vi "PID Setpoint Profile.vi"(4 "reinitialize? (F)":bool, 6 "dt (s)":dbl=-1.0 format="%.3f", 9 "setpoint profile":cluster{"time (s)":dbl, "setpoint":dbl}[](array[cluster]) {"setpoint" format="%.2f"; "time (s)" format="%.3f"}) -> (0 "dt out (s)":dbl format="%.3f", 1 "elapsed time (s)":dbl format="%.3f", 2 "profile complete?":bool, 3 "setpoint":dbl format="%.2f")   [LabVIEW 2017, in "NI_PID_pid.lvlib"]
doc: "Generates setpoint values over time in a control loop for ramp and soak types of control applications."
uses:
  <vilib>/addons/control/pid/NI_PID_pid.lvlib
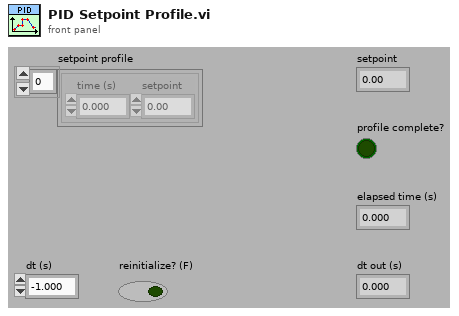
[diagram p1: front panel]
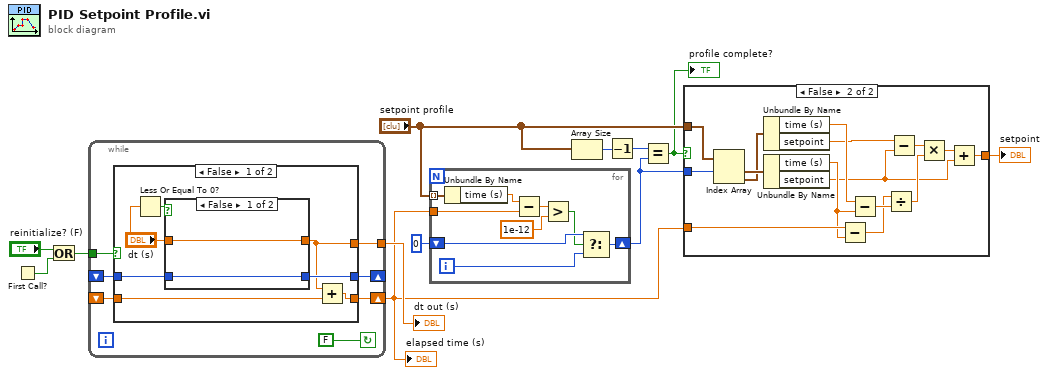
[diagram p0: block diagram]
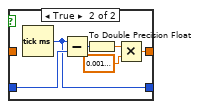
[diagram p2: hidden frame]
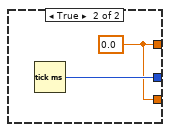
[diagram p3: hidden frame]
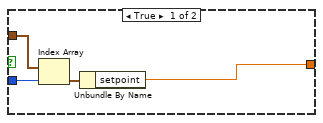
[diagram p4: hidden frame]
diagram:
  n1 = First Call?() -> (First Call?: T/F=w12:bool)
  n2 = Or(x="reinitialize? (F)", y=w12) -> (x .or. y?=w11:bool)
  n3 = while {
    tunnel: [w13] -> w2
    shift-left: _ -> [w16]
    shift-right: [w17] -> w1
    tunnel: w11 -> [w19]
    shift-left: _ -> [w14]
    shift-right: [w18] -> _
    stop <- FALSE continue-if-true
    n4 = case shown="False" w19 {
      tunnel: [w21 w36] -> w18
      tunnel: [w26 w35] -> w17
      tunnel: w16 -> [w25 _]
      tunnel: w14 -> [w22 _]
      tunnel: [w20 w35] -> w13
      frame False {
        n5 = Less Or Equal To 0?(x="dt (s)") -> (x <= 0?=w24:bool)
        n6 = case shown="False" w24 {
          tunnel: [w28 w31] -> w20
          tunnel: w22 -> [w27 w30]
          tunnel: [w27 w29] -> w21
          tunnel: "dt (s)" -> [w28 _]
          frame False {
          }
          frame True {
            n7 = Tick Count (ms)() -> (millisecond timer value=w29:u32)
            n8 = Subtract(x=w29, y=w30) -> (x-y=w33:u32)
            n9 = To Double Precision Float(number=w33) -> (double precision float=w32:dbl)
            n10 = Multiply(x=w32, y=0.0010000000474974513) -> (x*y=w31:dbl)
          }
        }
        n11 = Add(x=w20, y=w25) -> (x+y=w26:dbl)
      }
      frame True {
        w35 = 0.0
        n12 = Tick Count (ms)() -> (millisecond timer value=w36:u32)
      }
    }
  }
  "dt out (s)" <- w2
  "elapsed time (s)" <- w1
  n13 = for {
    tunnel: "setpoint profile" -> [w45] mode=indexing
    tunnel: w1 -> [w42]
    shift-right: [w44] -> w7
    shift-left: 0 -> [w41]
    i -> [w40]
    n14 = Unbundle By Name(w45) -> ("time (s)"=w43:dbl)
    n15 = Subtract(x=w43, y=w42) -> (x-y=w38:dbl)
    n16 = Greater?(x=w38, y=1e-12) -> (0:w39:bool)
    n17 = Select(t=w41, s=w39, f=w40) -> (s? t:f=w44:i32)
  }
  n18 = Array Size(array="setpoint profile") -> (size(s)=w10:i32)
  n19 = Decrement(x=w10) -> (x-1=w8:i32)
  n20 = Equal?(x=w8, y=w7) -> (x = y?=w3:bool)
  "profile complete?" <- w3
  n21 = case shown="False" w3 {
    tunnel: "setpoint profile" -> [w48 w62]
    tunnel: w7 -> [w47 w61]
    tunnel: [w46 w50] -> w6
    tunnel: w1 -> [_ w59]
    frame True {
      n22 = Index Array(array=w48, index=w47) -> (element=w49:cluster{"time (s)":dbl, "setpoint":dbl})
      n23 = Unbundle By Name(w49) -> ("setpoint"=w46:dbl)
    }
    frame False {
      n24 = Index Array(array=w62, index #1=w61) -> (element #1=w64:cluster{"time (s)":dbl, "setpoint":dbl}, element #2=w63:cluster{"time (s)":dbl, "setpoint":dbl})  [unwired: 1 in]
      n25 = Unbundle By Name(w63) -> ("time (s)"=w60:dbl, "setpoint"=w55:dbl)
      n26 = Unbundle By Name(w64) -> ("time (s)"=w58:dbl, "setpoint"=w51:dbl)
      n27 = Subtract(x=w59, y=w58) -> (x-y=w56:dbl)
      n28 = Subtract(x=w60, y=w58) -> (x-y=w57:dbl)
      n29 = Divide(x=w56, y=w57) -> (x/y=w53:dbl)
      n30 = Subtract(x=w55, y=w51) -> (x-y=w54:dbl)
      n31 = Multiply(x=w54, y=w53) -> (x*y=w52:dbl)
      n32 = Add(x=w52, y=w51) -> (x+y=w50:dbl)
    }
  }
  "setpoint" <- w6
